vi "BuildTestFromVI.vi"(8 "error in (no error)":errorcluster, 10 "VI Refnum":refnum<vi>, 11 "LVUnitTestBuilder in":refnum<class "LVUnitTestBuilder.lvclass">) -> (0 "error out":errorcluster, 2 "Test":refnum<class "Test.lvclass">, 3 "LVUnitTestBuilder out":refnum<class "LVUnitTestBuilder.lvclass">)   [LabVIEW 2019, in "LVUnitTestBuilder.lvclass"]
uses:
  LVUnitTestBuilder.lvclass
  Test/Test.lvclass
  TestCase/Fact/Fact.lvclass
  C:/Users/de200256/Code/neuperger/lvunit/Test/Test.lvclass
  <vilib>/ErrorRing/Error Ring.xnode
  <vilib>/Utility/error.llb/Error Cluster From Error Code.vi
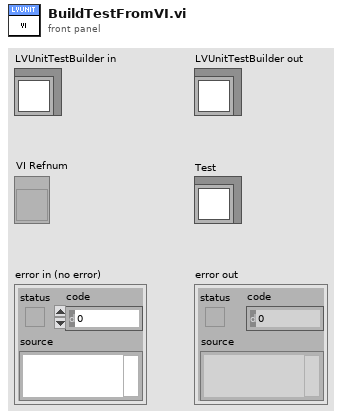
[diagram p1: front panel]
types:
  T1 = typedef "LVUnitTestBuilder.lvclass/Type.ctl" = enum16{"Unsupported", "Fact", "Theory"}
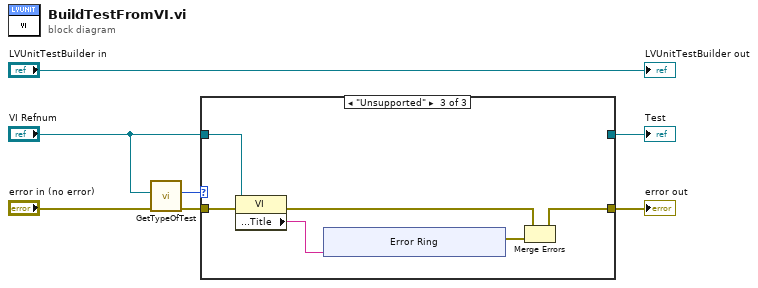
[diagram p0: block diagram]
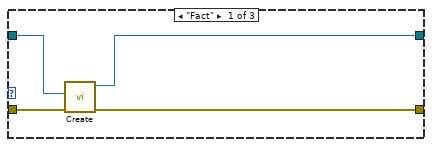
[diagram p2: hidden frame]
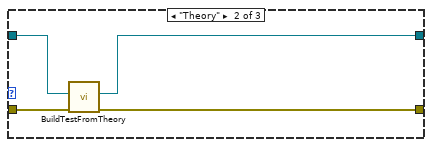
[diagram p3: hidden frame]
diagram:
  n1 = call "GetTypeOfTest.vi"("error in (no error)"="error in (no error)", "VI Refnum"="VI Refnum") -> ("error out"=w3:errorcluster, "Type"=w1:T1)  [unwired: 8 in]
  n2 = case shown="\"Unsupported\"" w1 {
    tunnel: [w11 w14 w19] -> w6
    tunnel: [w10 w12 _] -> w5
    tunnel: w3 -> [w9 w15 w20]
    tunnel: "VI Refnum" -> [w8 w13 w17]
    frame "Fact" {
      n3 = call "Create.vi"("error in (no error)"=w9, "VI Refnum"=w8) -> ("error out"=w11:errorcluster, "Fact"=w10:refnum<class "Fact.lvclass">)  [unwired: 8 in]
    }
    frame "Theory" {
      n4 = call "BuildTestFromTheory.vi"("error in (no error)"=w15, "VI Refnum"=w13) -> ("error out"=w14:errorcluster, "Test"=w12:refnum<class "Test.lvclass">)  [unwired: 8 in]
    }
    frame "Unsupported" {
      n5 = property class="VI"(reference=w17, error in=w20) -> (error out=w18:errorcluster, "Front Panel.Title"=w16:string)  [unwired: 1 out]
      n6 = xnode "Error Ring"("parameter 0"=w16) -> ("error out"=w21:errorcluster)
      n7 = Merge Errors(w18, w21) -> (w19:errorcluster)
    }
  }
  "error out" <- w6
  "Test" <- w5
  "LVUnitTestBuilder out" <- "LVUnitTestBuilder in"
